vi "Data Queue.vi"(7 "Action":T1(ring), 8 "error in (no error)":errorcluster, 11 "Data In":u16[][](array[numeric])) -> (0 "error out":errorcluster, 3 "Data Out":u16[][](array[numeric]))   [LabVIEW 2017]
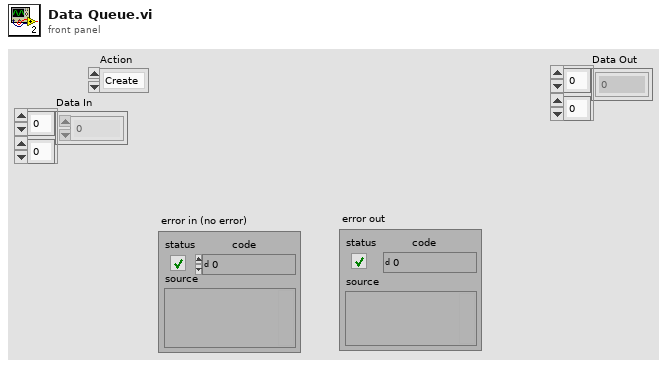
[diagram p1: front panel]
types:
  T1 = enum16{"Create", "Enqueue", "Dequeue", "Release"}
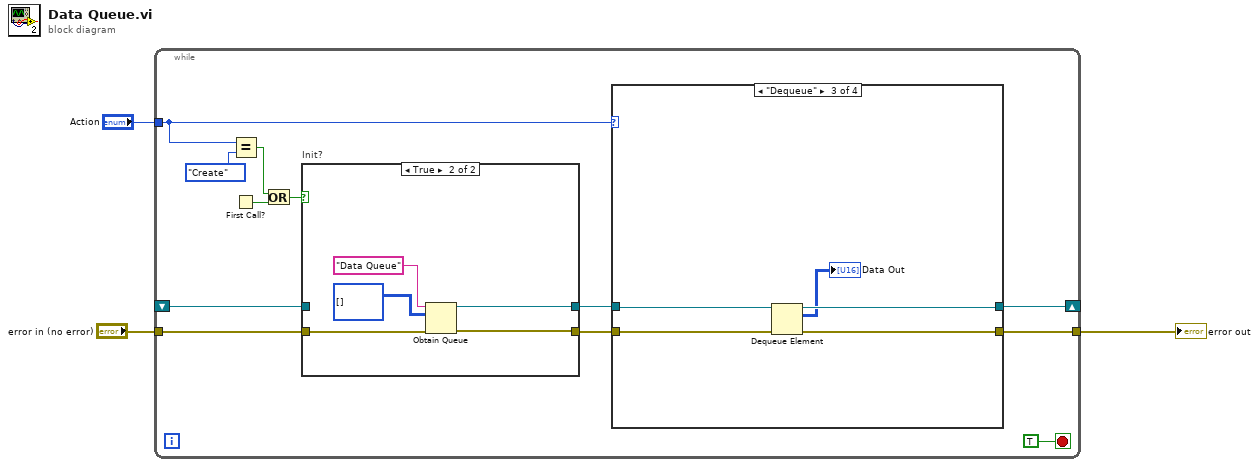
[diagram p0: block diagram]
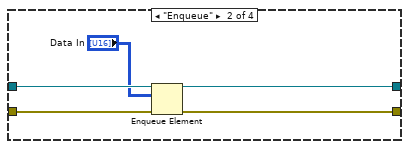
[diagram p4: hidden frame]
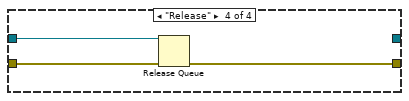
[diagram p5: hidden frame]
diagram:
  n1 = while {
    tunnel: "Action" -> [w14]
    tunnel: "error in (no error)" -> [w10]
    tunnel: [w8] -> w1
    shift-right: [w5] -> _
    shift-left: _ -> [w4]
    stop <- TRUE stop-if-true
    n2 = Equal?(x=w14, y=T1."Create") -> (x = y?=w12:bool)
    n3 = First Call?() -> (First Call?: T/F=w15:bool)
    n4 = Or(x=w12, y=w15) -> (x .or. y?=w11:bool)
    n5 = case "Init?" shown="True" w11 {
      tunnel: w10 -> [w17 w22]
      tunnel: [w17 w21] -> w9
      tunnel: [w16 w20] -> w6
      tunnel: w4 -> [w16 _]
      frame False {
      }
      frame True {
        n6 = Obtain Queue(name (unnamed)="Data Queue", element data type=u16[][] [] ("Data In"), error in (no error)=w22) -> (queue out=w20:refnum<queue>, error out=w21:errorcluster)  [unwired: 2 in, 1 out]
      }
    }
    n7 = case shown="\"Dequeue\"" w14 {
      tunnel: w9 -> [w24 w29 w34 w37]
      tunnel: [w24 w28 w31 w36] -> w8
      tunnel: w6 -> [w23 w26 w33 w35]
      tunnel: [w23 w27 w32 _] -> w5
      frame "Create", Default {
      }
      frame "Enqueue" {
        n8 = Enqueue Element(queue=w26, element="Data In", error in (no error)=w29) -> (queue out=w27:refnum<queue>, error out=w28:errorcluster)  [unwired: 2 out]
      }
      frame "Dequeue" {
        n9 = Dequeue Element(queue=w33, error in (no error)=w34) -> (queue out=w32:refnum<queue>, element=→"Data Out":u16[][], error out=w31:errorcluster)  [unwired: 2 out]
      }
      frame "Release" {
        n10 = Release Queue(queue=w35, error in (no error)=w37) -> (error out=w36:errorcluster)  [unwired: 1 in, 2 out]
      }
    }
  }
  "error out" <- w1
